vi "Abort Test Dequeue.vi"(8 "error in (no error)":errorcluster, 11 "ctlr queue":refnum<queue>) -> (0 "error out":errorcluster, 3 "abort?":bool)   [LabVIEW 2020]
uses:
  Controller Loop/Message and Data.ctl
  Parameter Class/IA Test Parameters.lvclass
  Controllers/Controller.lvclass
  Hardware/Sensors/Cameras/Camera.lvclass
  Hardware/Sensors/Force Sensors/Force Sensor.lvclass
  Hardware/Actuators/Servos/Servo.lvclass
  Hardware/Actuators/Switches/Switch.lvclass
  File Interfacing/Filename Structure.ctl
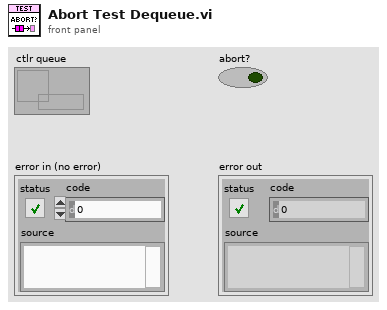
[diagram p1: front panel]
types:
  T1 = typedef "Message and Data.ctl" = cluster{"msg":string, "ia test param":refnum<class "IA Test Parameters.lvclass">, "controller type":refnum<class "Controller.lvclass">, "folder path":path, "file name":string, "file comments":string, "cam":refnum<class "Camera.lvclass">, "fs":refnum<class "Force Sensor.lvclass">, "servo":refnum<class "Servo.lvclass">, "switch":refnum<class "Switch.lvclass">, "filename struct":T2}
  T2 = typedef "Filename Structure.ctl" = enum16{"<nameYYYYMMDDi>", "<name>"}
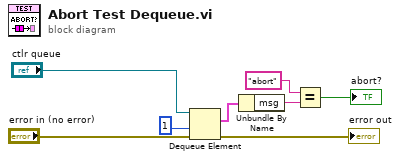
[diagram p0: block diagram]
diagram:
  n1 = Dequeue Element(queue="ctlr queue", timeout in ms (-1)=1, error in (no error)="error in (no error)") -> (element=w4:T1, error out=→"error out":errorcluster)  [unwired: 2 out]
  n2 = Unbundle By Name(w4) -> ("msg"=w3:string)
  n3 = Equal?(x="abort", y=w3) -> (x = y?=→"abort?":bool)
